vi "GenerateBodeStep.vi"(9 "Points/Decade":i32, 10 "Start Frequency":dbl, 11 "End Frequency":dbl) -> (3 "Log-Frequencies":dbl[](array[numeric]))   [LabVIEW 2019]
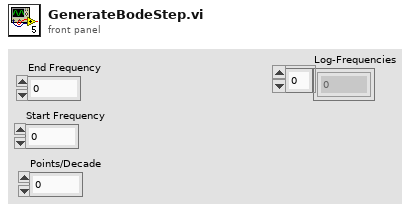
[diagram p1: front panel]
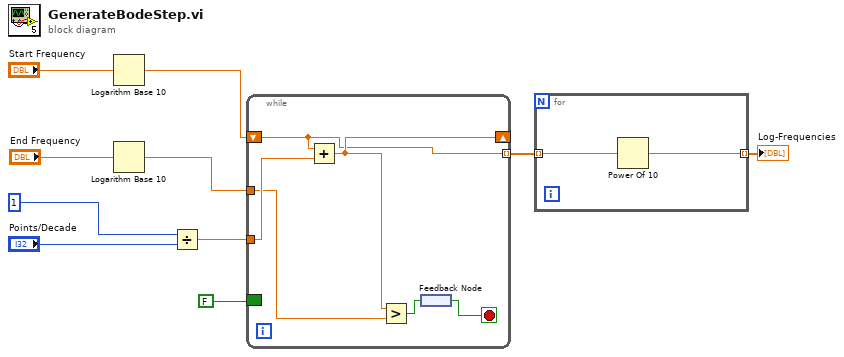
[diagram p0: block diagram]
diagram:
  n1 = Logarithm Base 10(1:"Start Frequency") -> (0:w6:dbl)
  n2 = Logarithm Base 10(1:"End Frequency") -> (0:w4:dbl)
  n3 = Divide(x=1, y="Points/Decade") -> (x/y=w5:dbl)
  n4 = while {
    tunnel: w5 -> [w16]
    tunnel: [w13] -> w3 mode=indexing
    tunnel: w4 -> [w15]
    shift-right: [w14] -> _
    shift-left: w6 -> [w13]
    border: FALSE -> [_]
    stop <- w11 stop-if-true
    n5 = Add(x=w13, y=w16) -> (x+y=w14:dbl)
    n6 = Greater?(x=w14, y=w15) -> (0:w12:bool)
    n7 = feedback-in #1(w12) -> ()
    n8 = feedback #1() -> (w11:bool)
  }
  n9 = for {
    tunnel: w3 -> [w18] mode=indexing
    tunnel: [w17] -> w2 mode=indexing
    n10 = Power Of 10(x=w18) -> (10^x=w17:dbl)
  }
  "Log-Frequencies" <- w2
